vi "GPIB Send.vi"(1 "Command String":string, 2 "Address":u16, 3 "VISA resource name":refnum<visa-resource-name>) -> (0 "Error":bool)   [LabVIEW 2017]
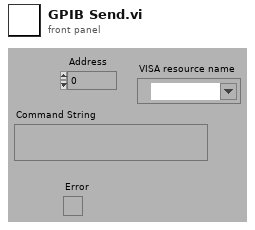
[diagram p1: front panel]
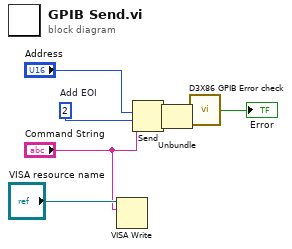
[diagram p0: block diagram]
diagram:
  w8 = u16 2  # Add EOI
  n1 = VISA Write(VISA resource name="VISA resource name", write buffer="Command String") -> ()  [unwired: 1 in, 3 out]
  n2 = Send(2:"Address", 3:w8, 5:"Command String") -> (6:w5:bool[], 8:w6:errorcluster)  [unwired: 2 in, 1 out]
  n3 = Unbundle(w6) -> ("code"=w3:i32)  [unwired: 2 out]
  n4 = call "D3X86 GPIB Error check.vi"("GPIB Error"=w3, "Status"=w5) -> ("Error"=→"Error":bool)
